vi "Process Current.vi"(8 "reference levels":T1={"high ref level"=90.0, "mid ref level"=75.0, "low ref level"=60.0, "ref units"=1} {"ref units" items=["absolute", "percent"]}, 9 "polarity (rising)":u16(ring)=1 items=["falling", "rising"], 10 "Channel Name":string, 11 "Waveform In":waveform(dbl)[](array[waveform])) -> (0 "Target Channel":waveform(dbl), 1 "Pulse Width":dbl, 2 "Quiescent":dbl, 3 "Slope":dbl, 4 "Pulse Peak Amplitude":dbl format="%.2g")   [LabVIEW 2019, in "Variant Parser.lvlib" / "Variant Parser.lvclass"]
uses:
  Library/Variant Parser.lvclass
  <vilib>/measure/mascope.llb/Amplitude and Levels 1 chan.vi
  <vilib>/measure/mascope.llb/Transition Measurements 1 chan.vi
  <vilib>/measure/NI_MAPro.lvlib
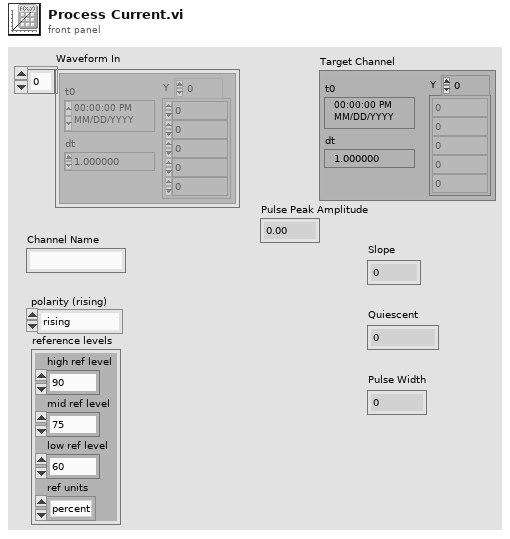
[diagram p1: front panel]
types:
  T1 = cluster{"high ref level":dbl, "mid ref level":dbl, "low ref level":dbl, "ref units":u16}
  T2 = cluster{"start time":dbl, "end time":dbl, "ref levels":cluster{"high ref level":dbl, "mid ref level":dbl, "low ref level":dbl, "ref units":u16}}
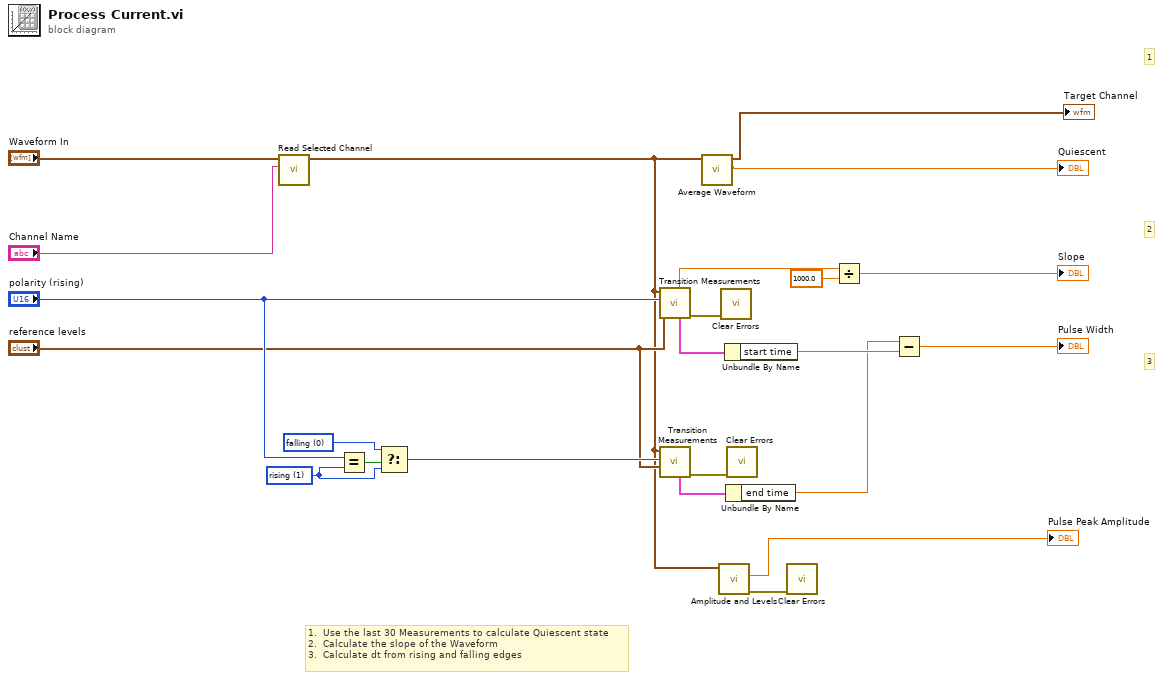
[diagram p0: block diagram]
diagram:
  w23 = u16 0 items=["falling", "rising"] ("polarity (rising)")
  w22 = u16 1 items=["falling", "rising"] ("polarity (rising)")
  # "1.  Use the last 30 Measurements to calculate Quiescent state\n2.  Calculate the slope of the Waveform\n3.  Calculate dt from rising and falling edges"
  # "3"
  # "2"
  # "1"
  n1 = call "Read Selected Channel.vi"("Channel Name"="Channel Name", "Waveform In"="Waveform In") -> ("Selected Channel"=w3:waveform(dbl))  [unwired: 9 in]
  n2 = Equal?(x="polarity (rising)", y=w22) -> (x = y?=w21:bool)
  n3 = Select(t=w23, s=w21, f=w22) -> (s? t:f=w19:u16)
  n4 = call-poly <vilib>:"Transition Measurements.vi"("reference levels"="reference levels", "polarity (rising)"="polarity (rising)", "signal in"=w3) -> ("error out"=w11:errorcluster, "measurement info"=w17:T2, "slope"=w18:dbl)  [unwired: 3 in, 3 out]
  n5 = call-poly <vilib>:"Transition Measurements.vi"("reference levels"="reference levels", "polarity (rising)"=w19, "signal in"=w3) -> ("error out"=w10:errorcluster, "measurement info"=w16:T2)  [unwired: 3 in, 4 out]
  n6 = call "Average Waveform.vi"("Channel in"=w3) -> ("Quiescent"=→"Quiescent":dbl, "Channel Out"=→"Target Channel":waveform(dbl))  [unwired: 9 in]
  n7 = call-poly <vilib>:"Amplitude and Levels.vi"("signal in"=w3) -> ("error out"=w7:errorcluster, "high state level"=→"Pulse Peak Amplitude":dbl)  [unwired: 7 in, 2 out]
  n8 = call <vilib>:"Clear Errors.vi"("error in (no error)"=w11) -> ()  [unwired: 5 in, 2 out]
  n9 = Unbundle By Name(w17) -> ("start time"=w15:dbl)
  n10 = Unbundle By Name(w16) -> ("end time"=w14:dbl)
  n11 = call <vilib>:"Clear Errors.vi"("error in (no error)"=w10) -> ()  [unwired: 5 in, 2 out]
  n12 = call <vilib>:"Clear Errors.vi"("error in (no error)"=w7) -> ()  [unwired: 5 in, 2 out]
  n13 = Divide(x=w18, y=1000.0) -> (x/y=→"Slope":dbl)
  n14 = Subtract(x=w14, y=w15) -> (x-y=→"Pulse Width":dbl)
